vi "get next Test Id.vi"(8 "error in (no error)":errorcluster, 11 "Norm in":refnum<class "Norm.lvclass">) -> (0 "error out":errorcluster, 2 "id":u32, 3 "Norm out":refnum<class "Norm.lvclass">)   [LabVIEW 2013, in "DatenKlassen.lvlib" / "Norm.lvclass"]
uses:
  Norm.lvclass
  Norm.lvclass/Norm.ctl
  Test/Test.lvclass
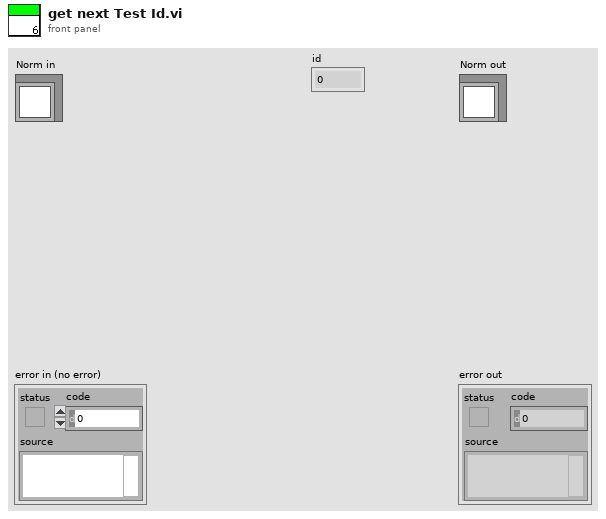
[diagram p1: front panel]
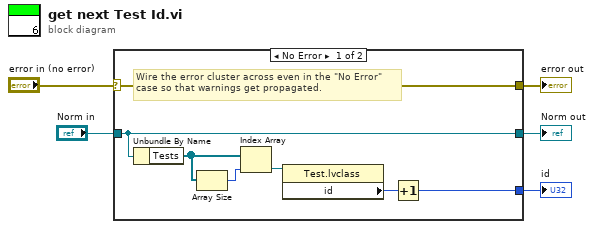
[diagram p0: block diagram]
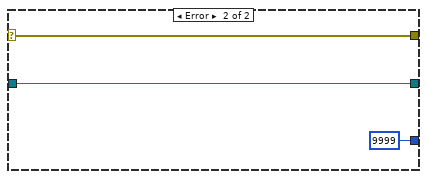
[diagram p2: hidden frame]
diagram:
  n1 = case shown="No Error" "error in (no error)" {
    selector: "error in (no error)" -> [w12 w15]
    tunnel: [w12 w15] -> w4
    tunnel: [w11 w14] -> w2
    tunnel: "Norm in" -> [w11 w14]
    tunnel: [w7 u32 9999 ("id")] -> w1
    frame No Error {
      # "Wire the error cluster across even in the \"No Error\"\ncase so that warnings get propagated."
      n2 = Unbundle By Name(w11) -> ("Tests"=w10:refnum<class "Test.lvclass">[])
      n3 = Array Size(array=w10) -> (size(s)=w9:i32)
      n4 = Index Array(array=w10, index=w9) -> (element=w8:refnum<class "Test.lvclass">)
      n5 = property class="Test.lvclass"(reference=w8) -> ("id"=w6:u32)  [unwired: 1 in, 2 out]
      n6 = Increment(x=w6) -> (x+1=w7:u32)
    }
    frame Error {
    }
  }
  "error out" <- w4
  "Norm out" <- w2
  "id" <- w1
